vi "Circle.vi"(8 "error in (no error)":errorcluster, 10 "target":refnum<class "pCircle.lvclass">, 11 "pCircle in":refnum<class "pCircle.lvclass">) -> (0 "error out":errorcluster, 3 "pCircle out":refnum<class "pCircle.lvclass">)   [LabVIEW 2017, in "pCircle.lvclass"]
uses:
  pCircle.lvclass
  C:/Users/fflores/Documents/LabVIEW-Open-Projects/LabIVEW OOP Design Patterns/Prototype Pattern/Shape Class/pShape.lvclass
  pCircle.lvclass/pCircle.ctl
  Shape Class/pShape.lvclass
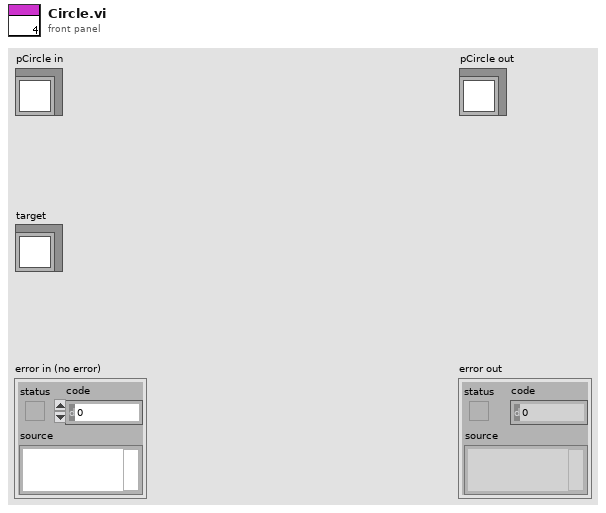
[diagram p1: front panel]
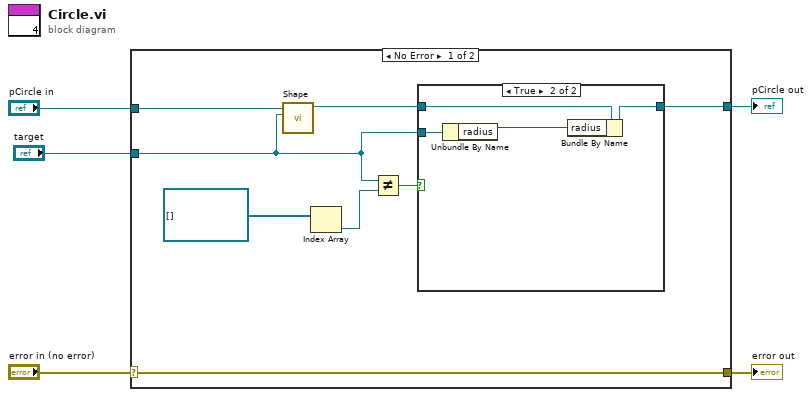
[diagram p0: block diagram]
diagram:
  n1 = case shown="No Error" "error in (no error)" {
    selector: "error in (no error)" -> [w13 w19]
    tunnel: [w13 w19] -> w4
    tunnel: [w9 w20] -> w2
    tunnel: "pCircle in" -> [w10 w20]
    tunnel: "target" -> [w7 _]
    frame No Error {
      n2 = call "Shape.vi"("pShape.lvclass"=w7, "pShape in"=w10) -> ("pShape out"=w8:refnum<class "pCircle.lvclass">)  [unwired: 8 in, 1 out]
      n3 = Index Array(array=refnum<class "pCircle.lvclass">[] []) -> (element=w12:refnum<class "pCircle.lvclass">)  [unwired: 1 in]
      n4 = Not Equal?(x=w7, y=w12) -> (x != y?=w6:bool)
      n5 = case shown="True" w6 {
        tunnel: [w14 w18] -> w9
        tunnel: w8 -> [w14 w17]
        tunnel: w7 -> [_ w16]
        frame False {
        }
        frame True {
          n6 = Unbundle By Name(w16) -> ("radius"=w15:i32)
          n7 = Bundle By Name(cluster=w17, "radius"=w15) -> (w18:refnum<class "pCircle.lvclass">)
        }
      }
    }
    frame Error {
      # "Wire the error cluster across even in the \"No Error\"\ncase so that warnings get propagated."
    }
  }
  "error out" <- w4
  "pCircle out" <- w2
